vi "FrontPanel_vs_BlockDia.vi"   [LabVIEW 2012]
uses:
  SubVIs/LVPresent_Globals.vi
panel:
  # "Front Panel vs. Block Diagram"
  # "The Front Panel:\n-adds buttons, switches, dials, numbers, decorations, etc.\n-is where the \"User interface\" is created\n-all graphs are viewed in the Front Panel."
  # "The Block Diagram:\n-where the actual code is composed \n-anything that is added in the front panel is shown on the block diagram\n-we will only be using the Block Diagram in this tutorial"
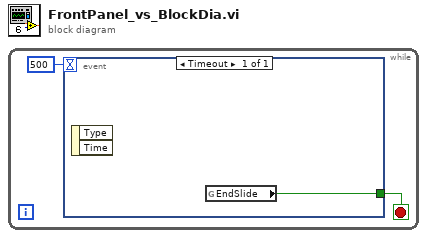
[diagram p0: block diagram]
diagram:
  n1 = while {
    stop <- w2 stop-if-true
    n2 = event shown="[0] Timeout" {
      selector: _ -> [_]
      dyn-events: _ -> [_]
      timeout: 500 -> [_]
      tunnel: [w3] -> w2
      event Timeout {
        n3 = event-data() -> ()  [unwired: 1 in, 2 out]
        n4 = global read "LVPresent_Globals.vi" "EndSlide"() -> (w3:bool)
      }
    }
  }
